vi "Display.vi"(2 "node":string, 3 "error in":errorcluster) -> (0 "error out":errorcluster)   [LabVIEW 2013]
doc: "This will nod the head."
uses:
  <vilib>/picture/picture.llb/imagedata.ctl
panel:
  out "2D Picture":picture
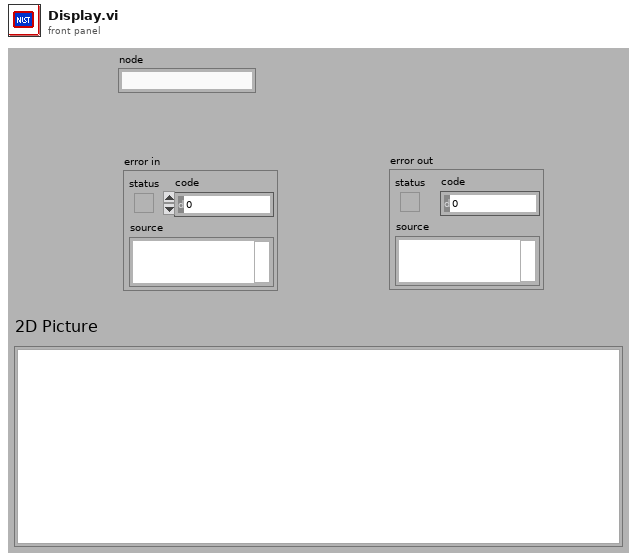
[diagram p1: front panel]
types:
  T1 = cluster{"Height":u32, "Width":u32, "is_bigendian?":u8, "Step":u32, "Data":u8[], "Encoding":string, "Frame ID":string}
  T2 = cluster{"left":i16, "top":i16, "right":i16, "bottom":i16}
  T3 = typedef "imagedata.ctl" = cluster{"image type":i32, "image depth":i32, "image":u8[], "mask":u8[], "colors":u32[], "Rectangle":cluster{"left":i16, "top":i16, "right":i16, "bottom":i16}}
  T4 = typedef "_ROSControl.ctl" = cluster{"topic port":u16, "Node":string, "topic":string, "type":string, "node port":u32, "error ":errorcluster, "Direction":T5, "APIs":string[]}
  T5 = typedef "_ROSDirection.ctl" = enum16{"Node", "Publisher", "Subscriber", "Service Client"}
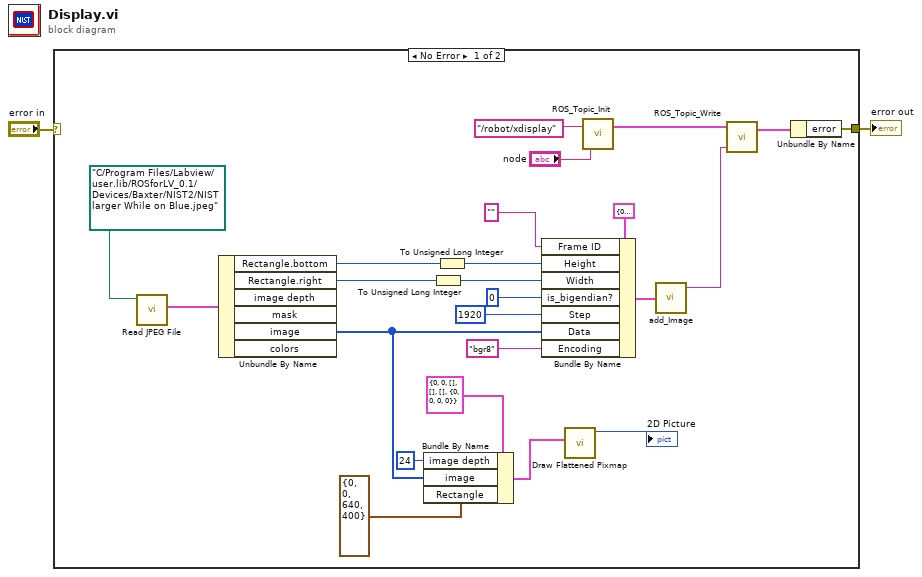
[diagram p0: block diagram]
diagram:
  n1 = case shown="No Error" "error in" {
    selector: "error in" -> [_ w27]
    tunnel: [w24 w27] -> w2
    frame No Error {
      n2 = call <vilib>:"Read JPEG File.vi"("path to JPEG file"=path "C:/Program Files/Labview/user.lib/ROSforLV_0.1/Devices/Baxter/NIST2/NIST larger While on Blue.jpeg") -> ("image data"=w6:T3)  [unwired: 8 in, 2 out]
      n3 = Unbundle By Name(w6) -> ("Rectangle.bottom"=w21:i16, "Rectangle.right"=w20:i16, "image"=w8:u8[])  [unwired: 3 out]
      n4 = Bundle By Name(cluster=T3 {"image type"=0, "image depth"=0, "image"=[], "mask"=[], "colors"=[], "Rectangle"={"left"=0, "top"=0, "right"=0, "bottom"=0}} ("image data"), "image depth"=24, "image"=w8, "Rectangle"=T2 {"left"=0, "top"=0, "right"=640, "bottom"=400}) -> (w11:T3)
      n5 = To Unsigned Long Integer(number=w20) -> (unsigned 32bit integer=w18:u32)
      n6 = To Unsigned Long Integer(number=w21) -> (unsigned 32bit integer=w19:u32)
      n7 = Bundle By Name(cluster=T1 {"Height"=0, "Width"=0, "is_bigendian?"=0, "Step"=0, "Data"=[], "Encoding"="", "Frame ID"=""} ("ROS Image"), "Frame ID"="" ("Header.Frame ID"), "Height"=w19, "Width"=w18, "is_bigendian?"=u8 0, "Step"=u32 1920, "Data"=w8, "Encoding"="bgr8") -> (w4:T1)
      n8 = call <vilib>:"Draw Flattened Pixmap.vi"("image data"=w11) -> ("new picture"=→"2D Picture":picture)  [unwired: 8 in]
      n9 = call "ROS_Topic_Init.vi"("node"="node", "topic"="/robot/xdisplay") -> ("ROS out"=w22:T4)  [unwired: 1 in]
      n10 = call "add_Image.vi"("ROS Image"=w4) -> ("msg out"=w3:string)  [unwired: 4 in]
      n11 = call "ROS_Topic_Write.vi"("Msg in"=w3, "ROS in"=w22) -> ("ROS out"=w25:T4)  [unwired: 2 in]
      n12 = Unbundle By Name(w25) -> ("error"=w24:errorcluster)
    }
    frame Error {
    }
  }
  "error out" <- w2
